vi "Write TopRef.vi"(8 "error in (no error)":errorcluster, 10 "TopRef":T1, 11 "UIActorTop2 in":refnum<class "UI_Top.lvclass">) -> (0 "error out":errorcluster, 3 "UIActorTop2 out":refnum<class "UI_Top.lvclass">)   [LabVIEW 2021, in "UI_Top.lvclass"]
uses:
  UI_Top.lvclass
  UI_Top.lvclass/UI_Top.ctl
  TopRef.ctl
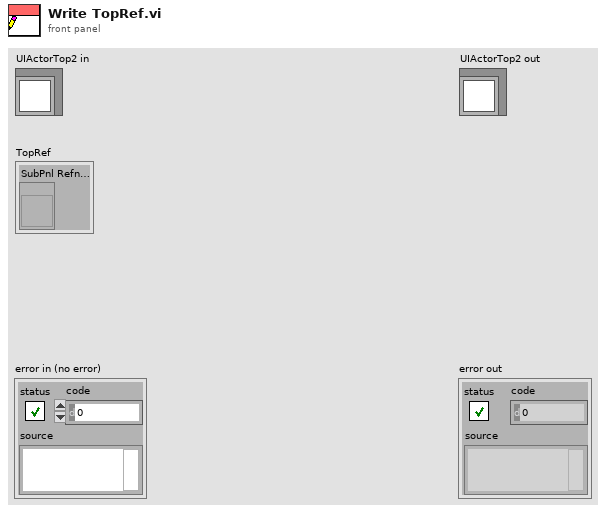
[diagram p1: front panel]
types:
  T1 = typedef "UI_Top.lvclass/TopRef.ctl" = cluster{"SubPnl Refnum":refnum<vi>}
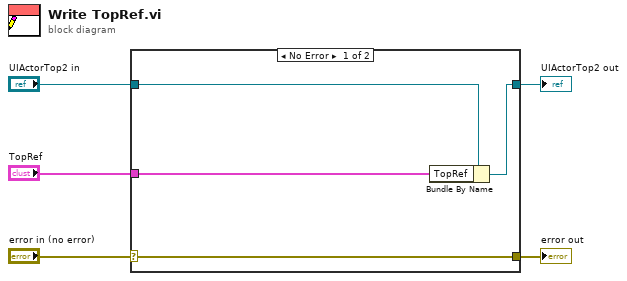
[diagram p0: block diagram]
diagram:
  n1 = case shown="No Error" "error in (no error)" {
    selector: "error in (no error)" -> [w9 w10]
    tunnel: [w9 w10] -> w4
    tunnel: [w7 w11] -> w2
    tunnel: "UIActorTop2 in" -> [w8 w11]
    tunnel: "TopRef" -> [w6 _]
    frame No Error {
      n2 = Bundle By Name(cluster=w8, "TopRef"=w6) -> (w7:refnum<class "UI_Top.lvclass">)
    }
    frame Error {
    }
  }
  "error out" <- w4
  "UIActorTop2 out" <- w2
